vi "Format RX data2.vi"(1 "Output Packet Array":i32[][](array[numeric])) -> (0 "new picture":picture)   [LabVIEW 2019]
uses:
  <vilib>/picture/picture.llb/Draw True-Color Pixmap.vi
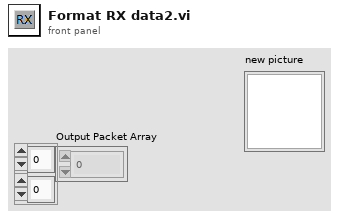
[diagram p1: front panel]
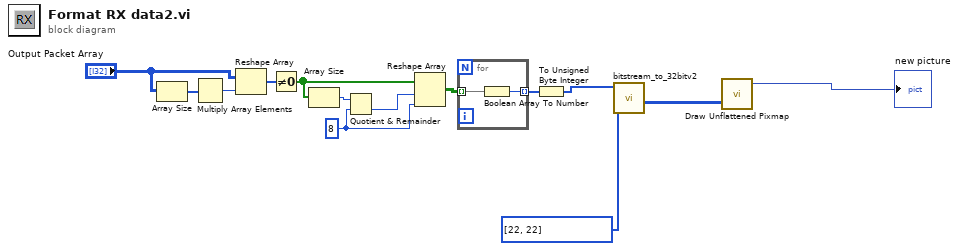
[diagram p0: block diagram]
diagram:
  w12 = 8 ("dimension size")
  n1 = Array Size(array="Output Packet Array") -> (size(s)=w6:i32[])
  n2 = Multiply Array Elements(1:w6) -> (0:w8:i32)
  n3 = Reshape Array "Reshape Array"("Output Packet Array", w8) -> (w9:i32[])
  n4 = Not Equal To 0?(x=w9) -> (x != 0?=w10:bool[])
  n5 = Array Size(array=w10) -> (size(s)=w11:i32)
  n6 = Quotient & Remainder(x=w11, y=w12) -> (floor(x/y)=w5:i32)  [unwired: 1 out]
  n7 = Reshape Array(w10, w5, w12) -> (w13:bool[][])
  n8 = for {
    tunnel: w13 -> [w16] mode=indexing
    tunnel: [w15] -> w14 mode=indexing
    n9 = Boolean Array To Number(Boolean array=w16) -> (number=w15:u32)
  }
  n10 = To Unsigned Byte Integer(number=w14) -> (unsigned 8bit integer=w4:u8[])
  n11 = call "bitstream_to_32bitv2.vi"("JPG Size"=i32[] [22, 22], "Bitstream Input"=w4) -> ("2D JPG Array"=w3:u32[][])  [unwired: 8 in, 1 out]
  n12 = call-poly <vilib>:"Draw Unflattened Pixmap.vi"("data (RGB format)"=w3) -> ("new picture"=→"new picture":picture)  [unwired: 8 in]
